vi "cross_link_to_excel.vi"(8 "error in (no error)":errorcluster, 9 "position (excel).row":i32, 10 "position (excel).column":i32, 11 "boc_data":sgl[][](array[numeric])) -> (0 "error out":errorcluster)   [LabVIEW 2017]
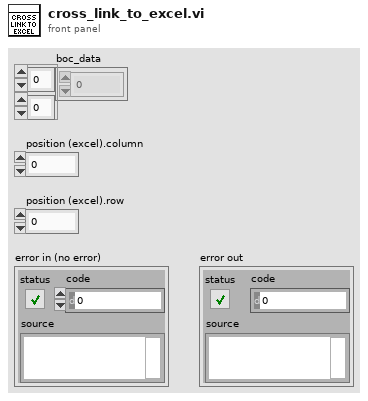
[diagram p1: front panel]
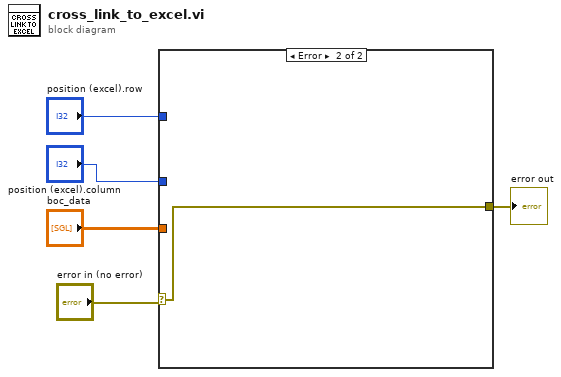
[diagram p0: block diagram]
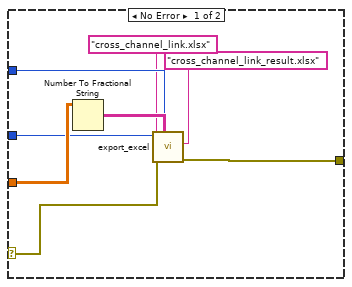
[diagram p2: hidden frame]
diagram:
  n1 = case shown="Error" "error in (no error)" {
    selector: "error in (no error)" -> [w6 w14]
    tunnel: [w13 w14] -> w5
    tunnel: "boc_data" -> [w11 _]
    tunnel: "position (excel).column" -> [w10 _]
    tunnel: "position (excel).row" -> [w9 _]
    frame No Error {
      n2 = Number To Fractional String(number=w11) -> (F-format string=w12:string[][])  [unwired: 3 in]
      n3 = call "export_excel.vi"("table"=w12, "position (excel).row"=w9, "error in (no error)"=w6, "template_filename"="cross_channel_link.xlsx", "result_filename"="cross_channel_link_result.xlsx", "position (excel).column"=w10) -> ("error out"=w13:errorcluster)  [unwired: 5 in]
    }
    frame Error {
    }
  }
  "error out" <- w5
